vi "ReadFPY.vi"(8 "error in (no error)":errorcluster) -> (0 "error out":errorcluster, 1 "FPY%":dbl, 2 "fail":i32, 3 "pass":i32, 5 "total":i32)   [LabVIEW 2013]
uses:
  <vilib>/Utility/file.llb/Read From Spreadsheet File (string).vi
panel:
  out "all rows":string[][](array[string])
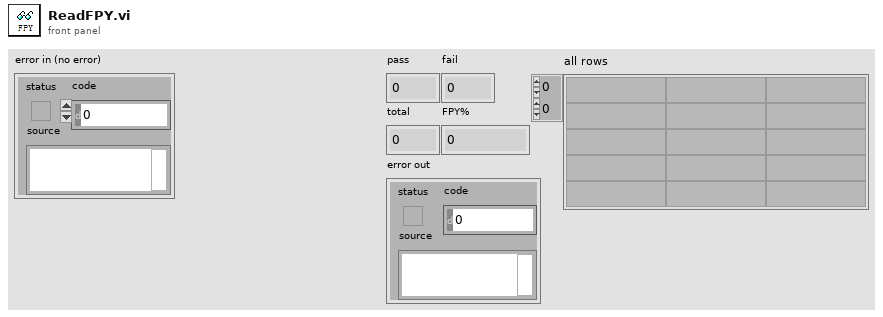
[diagram p1: front panel]
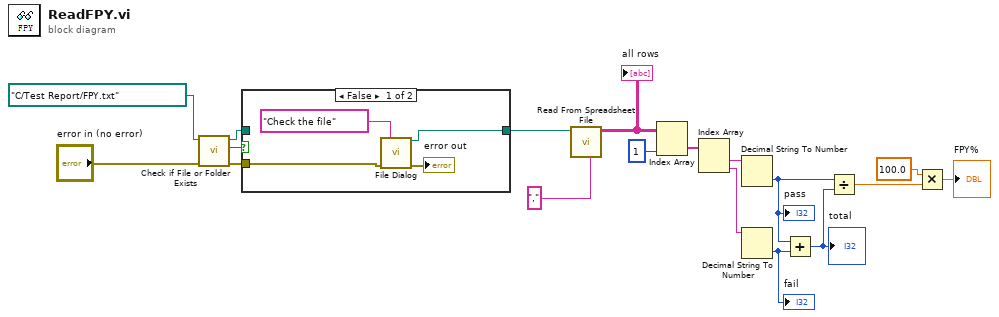
[diagram p0: block diagram]
diagram:
  n1 = call <vilib>:"Check if File or Folder Exists.vi"("error in (no error)"="error in (no error)", "path"=path "C:/Test Report/FPY.txt" ("start path")) -> ("error out"=w7:errorcluster, "file or folder exists?"=w17:bool, "dup path"=w16:path)  [unwired: 7 in]
  n2 = case shown="False" w17 {
    tunnel: w16 -> [_ w23]
    tunnel: [w22 w23] -> w15
    tunnel: w7 -> [w20 _]
    frame False {
      n3 = call "File Dialog"("prompt"="Check the file", "error in"=w20) -> ("selected path"=w22:path, "error out"=→"error out":errorcluster)  [unwired: 10 in, 2 out]
    }
    frame True {
    }
  }
  n4 = call-poly <vilib>:"Read From Spreadsheet File.vi"("delimiter (\\t)"="," ("delimiter (\\t)"), "file path (dialog if empty)"=w15) -> ("all rows"=w9:string[][])  [unwired: 5 in, 4 out]
  "all rows" <- w9
  n5 = Index Array(array=w9, index (col)=1 ("disabled index (col)")) -> (element=w12:string[])  [unwired: 1 in]
  n6 = Index Array(array=w12) -> (element #1=w11:string, element #2=w10:string)  [unwired: 2 in]
  n7 = Decimal String To Number(string=w11) -> (number=w5:i32)  [unwired: 2 in, 1 out]
  "pass" <- w5
  n8 = Decimal String To Number(string=w10) -> (number=w6:i32)  [unwired: 2 in, 1 out]
  "fail" <- w6
  n9 = Add(x=w5, y=w6) -> (x+y=w4:i32)
  "total" <- w4
  n10 = Divide(x=w5, y=w4) -> (x/y=w3:dbl)
  n11 = Multiply(x=100.0, y=w3) -> (x*y=→"FPY%":dbl)
